vi "kronenring.vi"(10 "Height":sgl, 11 "Radius":sgl) -> (0 "error out":errorcluster, 3 "Scene Object Out":refnum<vi>)   [LabVIEW 2014]
uses:
  <vilib>/picture/3D Picture Control/Object/Create Object (name).vi
  <vilib>/picture/3D Picture Control/Object/Create Object (drawable).vi
  <vilib>/picture/3D Picture Control/Object/Add Object (no reference).vi
  <vilib>/picture/3D Picture Control/NI_3D Picture Control.lvlib
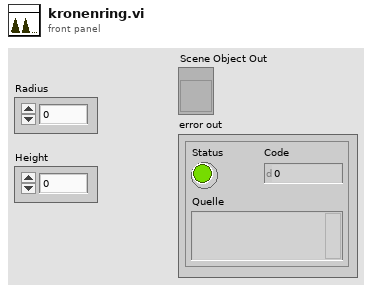
[diagram p1: front panel]
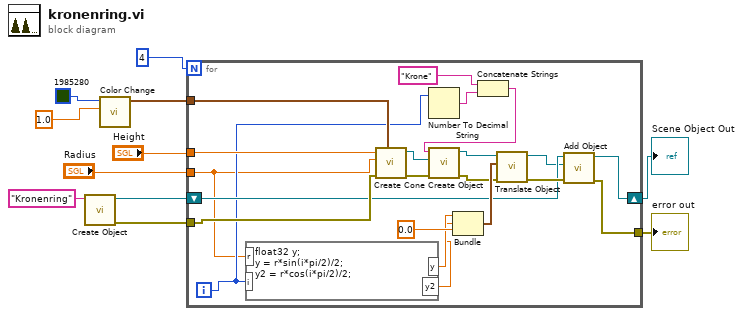
[diagram p0: block diagram]
diagram:
  n1 = call-poly <vilib>:"Create Object.vi"("Name"="Kronenring") -> ("error out"=w7:errorcluster, "Scene:New Object"=w8:refnum<vi>)  [unwired: 9 in]
  n2 = call <vilib>:"Color Change.vi"("Alpha"=1.0, "Color"=u32 1985280) -> ("RGBA"=w3:cluster{"R":sgl, "G":sgl, "B":sgl, "A":sgl})  [unwired: 9 in]
  n3 = for {
    N: 4 -> [_]
    tunnel: "Height" -> [w28]
    tunnel: "Radius" -> [w12]
    tunnel: w7 -> [w25]
    tunnel: w3 -> [w24]
    tunnel: [w17] -> w1
    shift-right: [w18] -> w2
    shift-left: w8 -> [w20]
    i -> [w16]
    n4 = formula code="float32 y;\ny = r*sin(i*pi/2)/2;\ny2 = r*cos(i*pi/2)/2;"("i"=w16, "r"=w12) -> ("y"=w31:sgl, "y2"=w30:dbl)
    n5 = call <vilib>:"Create Cone.vi"("Color"=w24, "error in (no error)"=w25, "Radius"=w12, "Height"=w28) -> ("error out"=w26:errorcluster, "New Cone Refnum"=w27:refnum<vi>)  [unwired: 6 in]
    n6 = Number To Decimal String(number=w16) -> (decimal integer string=w14:string)  [unwired: 1 in]
    n7 = Bundle(w31, "y2"=w30, "Radius"=sgl 0.0) -> (w29:cluster{sgl, "y2":dbl, "Radius":sgl})  [unwired: 1 in]
    n8 = Concatenate Strings("Krone" ("Name"), w14) -> (w13:string)
    n9 = call-poly <vilib>:"Create Object.vi"("error in (no error)"=w26, "Geometry"=w27, "Name"=w13) -> ("error out"=w22:errorcluster, "Scene:New Object"=w23:refnum<vi>)  [unwired: 7 in]
    n10 = call <vilib>:"Translate Object.vi"("error in (no error)"=w22, "Translation"=w29, "Scene.Object In"=w23) -> ("error out"=w21:errorcluster, "Scene.Object Out"=w19:refnum<vi>)  [unwired: 7 in]
    n11 = call-poly <vilib>:"Add Object.vi"("error in (no error)"=w21, "New Object In"=w19, "Scene Object In"=w20) -> ("error out"=w17:errorcluster, "Scene Object Out"=w18:refnum<vi>)  [unwired: 7 in]
  }
  "Scene Object Out" <- w2
  "error out" <- w1
